vi "MCC 172 Noise.vi"() -> ()   [LabVIEW 2018]
uses:
  <vilib>/addons/_NISVFA/_Shared subVIs/Controls/svc_Window.ctl
  <vilib>/Analysis/5stat.llb/RMS (DBL).vi
  <vilib>/addons/Sound and Vibration/svt_Single Tone Measurements/SVT Idle Channel Noise (Time) (1 Ch).vi
  <vilib>/addons/_NISVFA/_Baseband FFT/SVFA Power Spectral Density (1 Ch).vi
  <vilib>/addons/_NISVFA/_Baseband FFT/SVFA Power Spectrum (1 Ch).vi
  <vilib>/addons/Sound and Vibration/svt_Single Tone Measurements/SoundVib_SingleTone.lvlib
  <vilib>/Analysis/NI_AALBase.lvlib
  <vilib>/Analysis/NI_AALPro.lvlib
  <vilib>/gmath/NI_Gmath.lvlib
panel:
  in  "?":bool
  in  "# of Averaging":u32=1
  in  "Tab Control":enum32{"Setup", "Plots"}(tab)
  in  "IEPE Power":bool
  out "Actual Sampling Rate":dbl
  in  "Desired Sampling Rate":dbl=51200.0
  in  "Server IP Address":string
  in  "Channel":u8
  out "averaging parameters":T1={"averaging mode"=enum."RMS averaging", "weighting mode"=enum."Linear", "number of averages"=1, "linear mode"=enum."Auto restart"} {"number of averages" min=1 step=1}
  out "Data":T2={"SVT"={"Noise (BW)"=6.638588448604977e-06, "SNR [dB]"=114.52750191336867, "Avg Noise Density"=8.304726164455459e-08, "Maximum Spur"={"Frequency"=10.6, "Spur Level"=3.655230318410738e-07}}, "Max Data"=-9.28286463022232e-05, "Data Range"=6.53464812785387e-05, "Mean(Offset)"=-0.00012652362230801374, "StdDev (Noise)"=7.540583269192075e-06, "RMS Value"=0.00012674812231162398, "Spread Value"=0.0}
  out "error out":errorcluster
  out "frequency range":T3={"start frequency"=10.0, "stop frequency"=6400.0} {"stop frequency" format="%.2f"; "start frequency" format="%.2f"}
  out "dt":dbl=7.8125e-05
  in  "Samples to read":u32=51200
  out "FFT Plot":cluster{"f0":dbl, "df":dbl, "magnitude":dbl[]}(graph)={"f0"=0.0, "df"=0.2, "magnitude"=[]}
  out "Histogram":dynamicdata(graph)
  out "Noise Density":cluster{"f0":dbl, "df":dbl, "magnitude":dbl[]}(graph)={"f0"=0.0, "df"=0.2, "magnitude"=[]}
  out "AI Data":waveform(dbl)(graph)
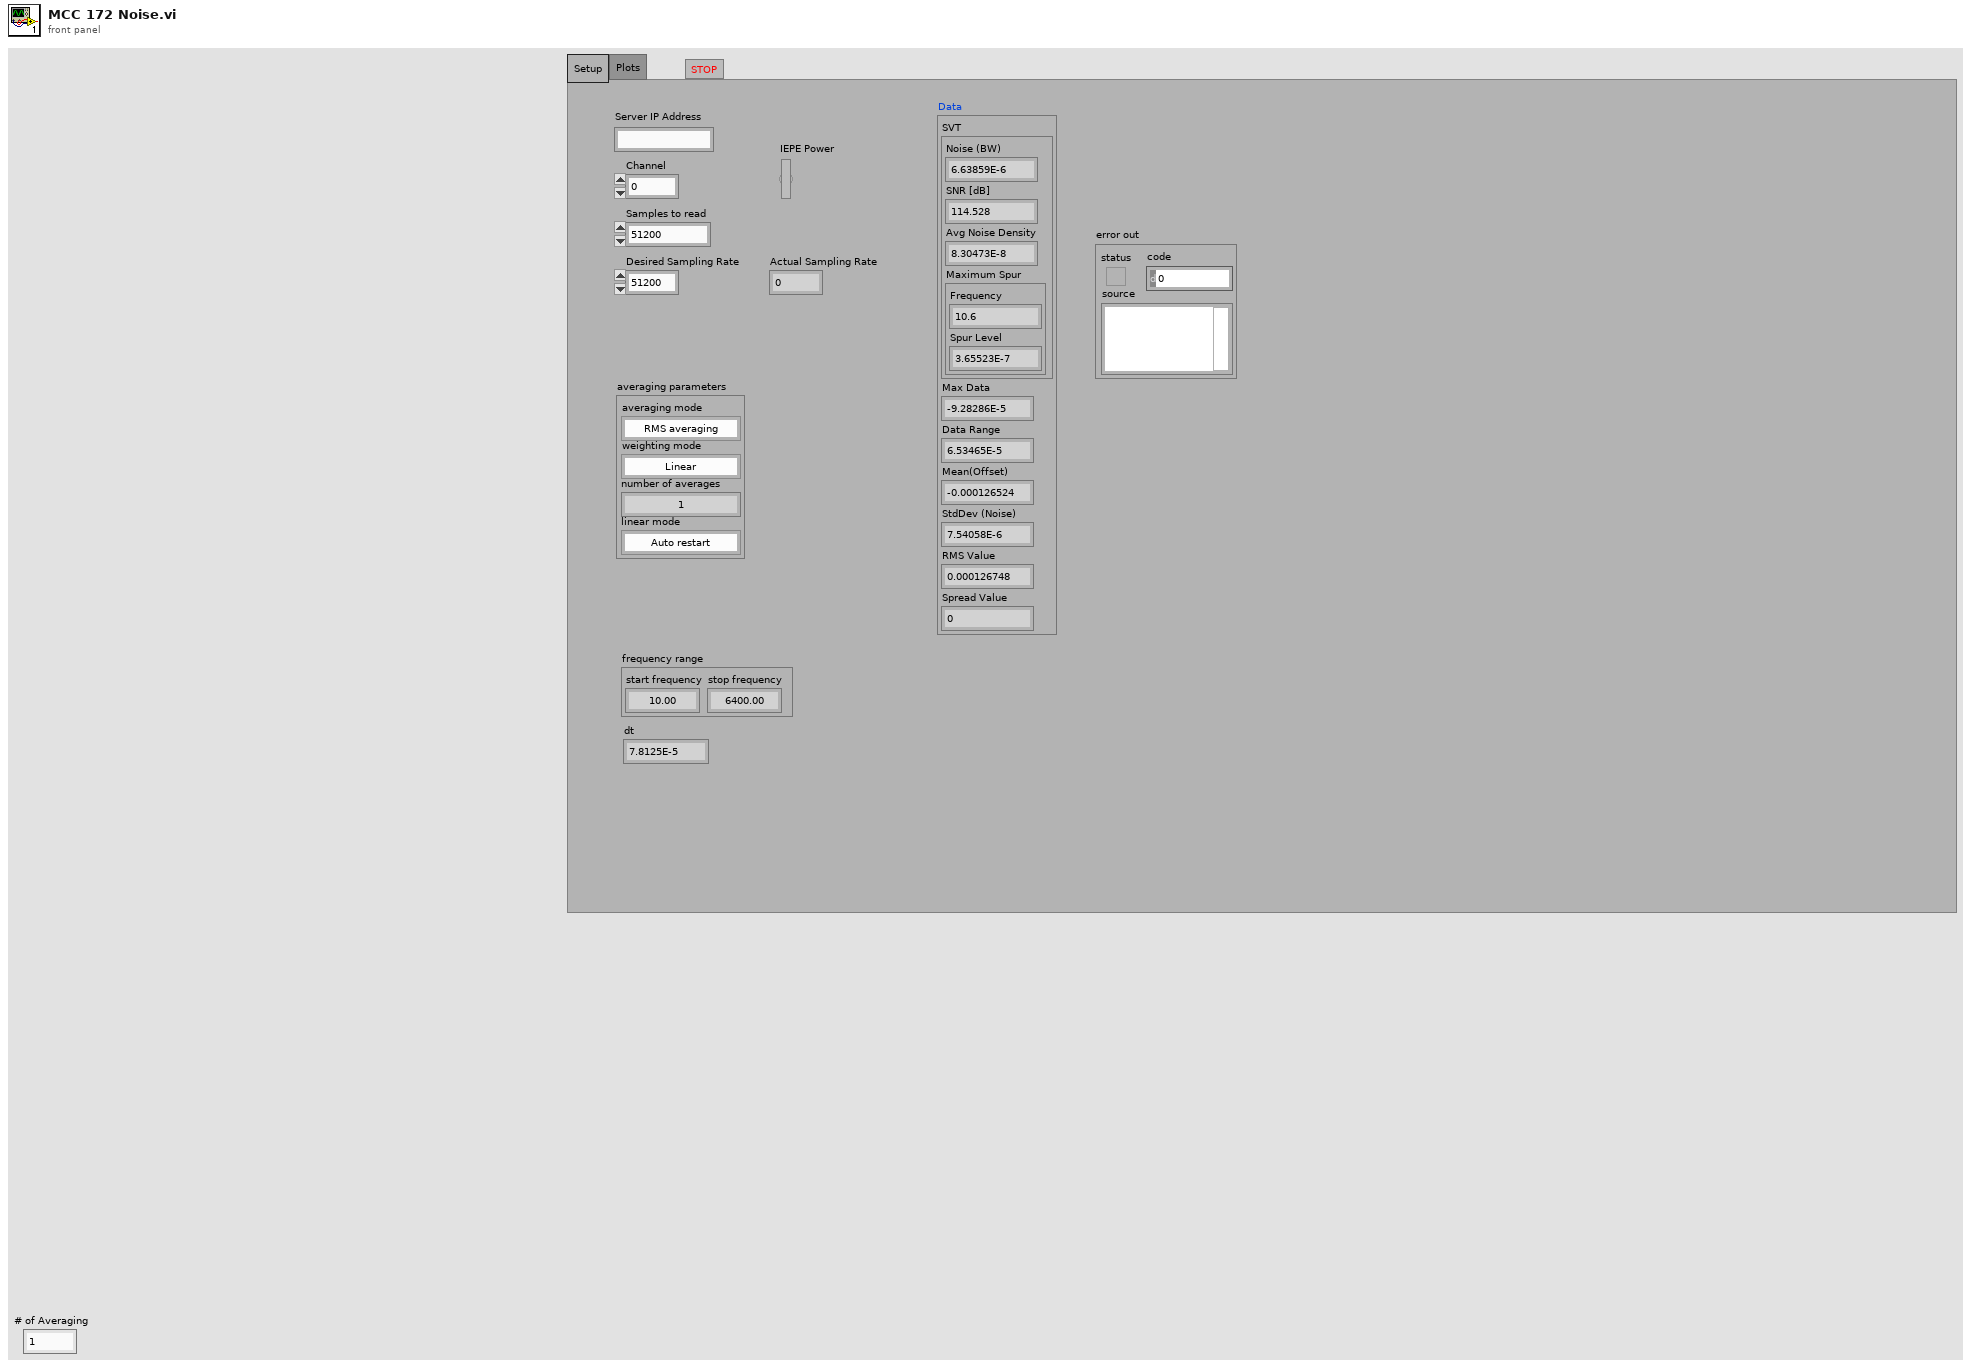
[diagram p1: front panel]
types:
  T1 = cluster{"averaging mode":enum16{"No averaging", "Vector averaging", "RMS averaging", "Peak hold"}, "weighting mode":enum16{"Linear", "Exponential"}, "number of averages":u32, "linear mode":enum16{"One shot", "Auto restart"}}
  T2 = cluster{"SVT":cluster{"Noise (BW)":dbl, "SNR [dB]":dbl, "Avg Noise Density":dbl, "Maximum Spur":cluster{"Frequency":dbl, "Spur Level":dbl}}, "Max Data":dbl, "Data Range":dbl, "Mean(Offset)":dbl, "StdDev (Noise)":dbl, "RMS Value":dbl, "Spread Value":dbl}
  T3 = cluster{"start frequency":dbl, "stop frequency":dbl}
  T4 = enum16{"No averaging", "Vector averaging", "RMS averaging", "Peak hold"}
  T5 = cluster{"idle channel noise units":enum16{"dB", "EU^2 rms"}}
  T6 = typedef "svc_Window.ctl" = u32
  T7 = cluster{dbl, "SNR [dB]":dbl, "average noise level [EU / sqrt(Hz)]":dbl, "maximum spur [EU rms]":cluster{"frequency":dbl, "value":dbl}}
  T8 = cluster{cluster{dbl, "SNR [dB]":dbl, "average noise level [EU / sqrt(Hz)]":dbl, "maximum spur [EU rms]":cluster{"frequency":dbl, "value":dbl}}, dbl, dbl, "mean":dbl, "standard deviation":dbl, "rms value":dbl, "spread value":dbl}
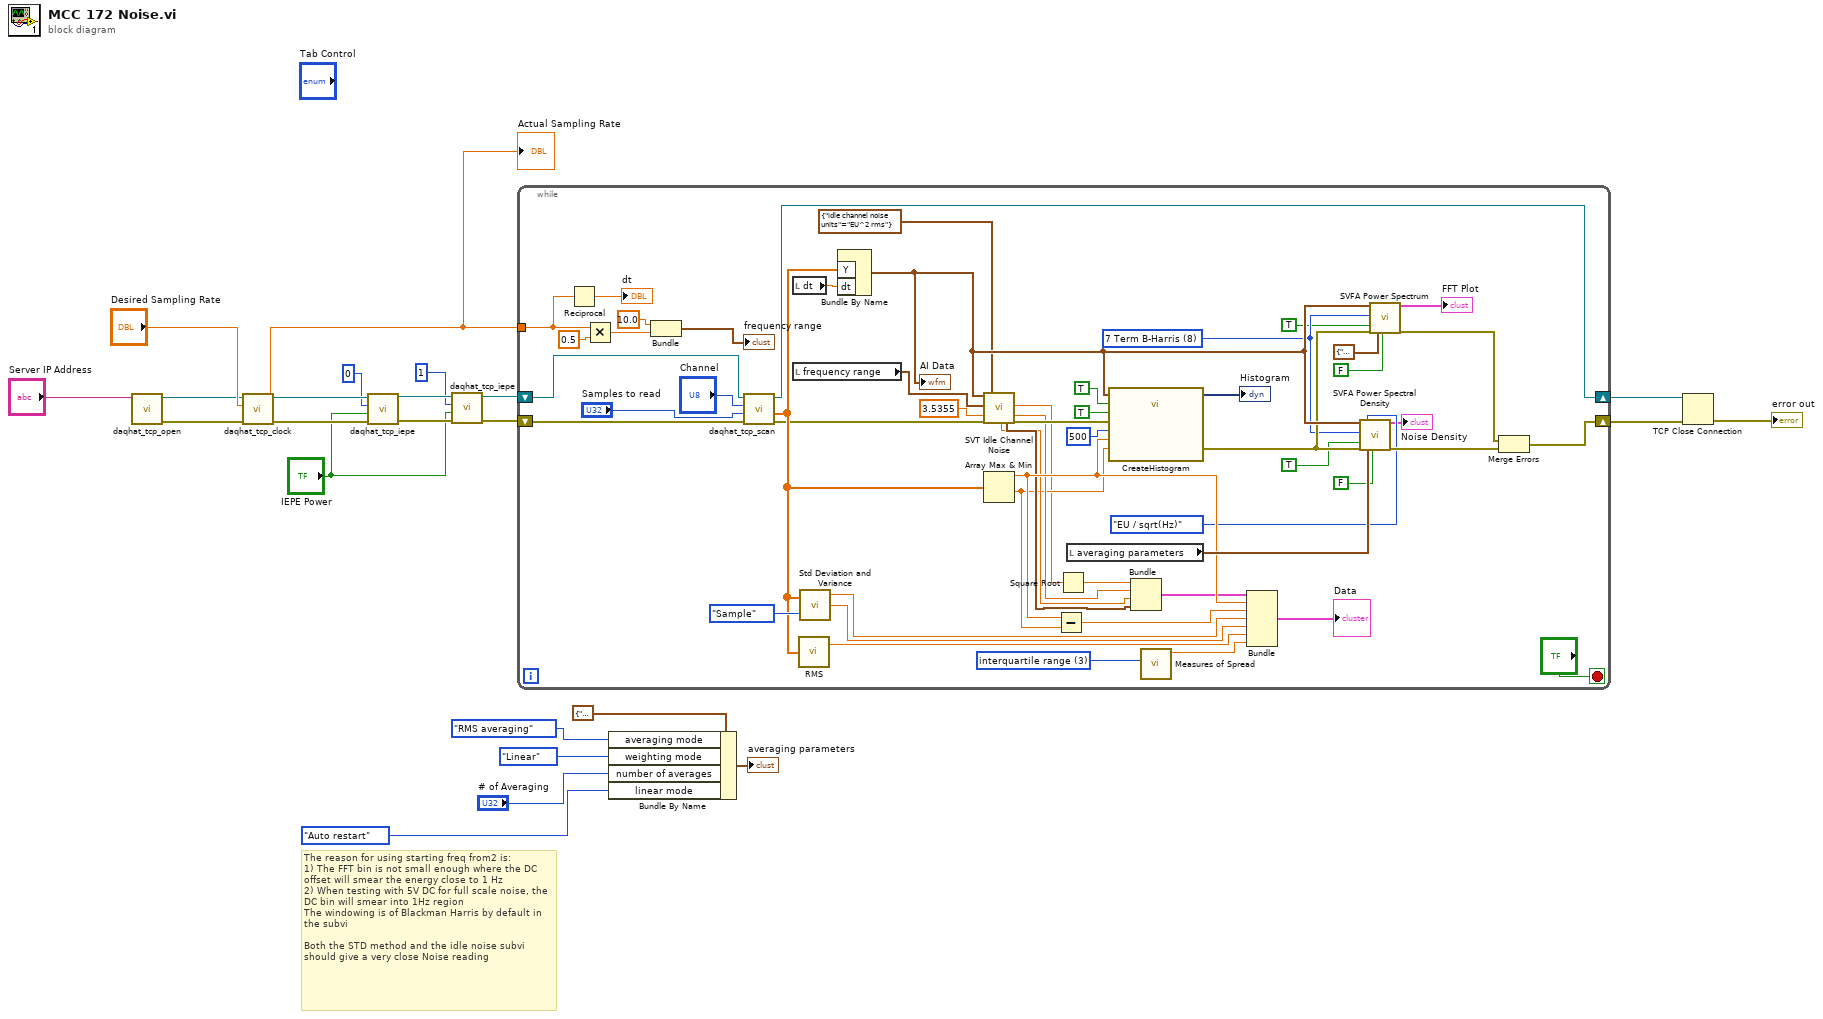
[diagram p0: block diagram]
diagram:
  # "The reason for using starting freq from2 is:\n1) The FFT bin is not small enough where the DC offset will smear the energy close to 1 Hz\n2) When testing with 5V DC for full scale noise, the DC bin will smear into 1Hz region\nThe windowing is of Blackman Harris by default in the subvi\n\nBoth the STD method and the idle noise subvi should give a very close Noise reading"
  n1 = call "daqhat_tcp_open.vi"("Server IP Address"="Server IP Address") -> ("error out"=w11:errorcluster, "TCP Network Connection out"=w10:refnum<k5>)  [unwired: 9 in]
  n2 = call "daqhat_tcp_clock.vi"("error in (no error)"=w11, "Desired frequency"="Desired Sampling Rate", "TCP network connection in"=w10) -> ("error out"=w8:errorcluster, "Set frequency"=w20:dbl, "TCP Network Connection out"=w9:refnum<k5>)  [unwired: 6 in]
  "Actual Sampling Rate" <- w20
  n3 = call "daqhat_tcp_iepe.vi"("error in (no error)"=w8, "IEPE Power"="IEPE Power", "Channel"=0, "TCP network connection in"=w9) -> ("error out"=w4:errorcluster, "TCP Network Connection out"=w3:refnum<k5>)  [unwired: 6 in]
  n4 = call "daqhat_tcp_iepe.vi"("error in (no error)"=w4, "IEPE Power"="IEPE Power", "Channel"=1, "TCP network connection in"=w3) -> ("error out"=w5:errorcluster, "TCP Network Connection out"=w6:refnum<k5>)  [unwired: 6 in]
  n5 = while {
    shift-right: [w37] -> w21
    shift-left: w5 -> [w42]
    shift-right: [w38] -> w23
    shift-left: w6 -> [w41]
    tunnel: w20 -> [w24]
    stop <- "?" stop-if-true
    w53 = T6 8 items=["None"=0, "Hanning"=1, "Hamming"=2, "Blackman-Harris"=3, "Exact Blackman"=4, "Blackman"=5, "Flat Top"=6, "4 Term B-Harris "=7, "7 Term B-Harris"=8, "Low Sidelobe"=9, "Force"=64, "Exponential"=65, "Blackman Nuttall"=11, "Triangle"=30, "Bartlett-Hanning"=31, "Bohman"=32, "Parzen"=33, "Welch"=34, "Kaiser"=60, "Dolph-Chebyshev"=61, "Gaussian"=62] ("window")
    w46 = 3 items=["standard deviation", "range", "mean absolute deviation", "interquartile range"] ("type")
    n6 = Reciprocal(x=w24) -> (1/x=→"dt":dbl)
    n7 = Multiply(x=w24, y=0.5) -> (x*y=w28:dbl)
    n8 = Bundle(10.0, w28) -> (→"frequency range":cluster{dbl, dbl})  [unwired: 1 in]
    n9 = call "daqhat_tcp_scan.vi"("error in (no error)"=w42, "Sample count"="Samples to read", "Analog channel"="Channel", "TCP network connection in"=w41) -> ("error out"=w39:errorcluster, "Sample data"=w40:dbl[], "TCP Network Connection out"=w38:refnum<k5>)  [unwired: 4 in, 1 out]
    n10 = local read "dt"() -> (w72:dbl)
    n11 = local read "frequency range"() -> (w73:T3)
    n12 = call-poly <vilib>:"RMS.vi"("X"=w40) -> ("rms value"=w68:dbl)  [unwired: 1 out]
    n13 = call <vilib>:"Std Deviation and Variance.vi"("X"=w40, "Weighting (Sample)"=enum16{"Sample", "Population"}."Sample") -> ("mean"=w66:dbl, "standard deviation"=w67:dbl)  [unwired: 1 out]
    n14 = Bundle By Name("Y"=w40, "dt"=w72) -> (w77:waveform(dbl))  [unwired: 1 in]
    "AI Data" <- w77
    n15 = call-poly <vilib>:"SVT Idle Channel Noise.vi"("scaled signal [EU]"=w77, "frequency range"=w73, "full-scale level [EU rms]"=3.5355, "error in (no error)"=w39, "desired units"=T5 {"idle channel noise units"=enum."EU^2 rms"}) -> ("average noise level [EU / sqrt(Hz)]"=w61:dbl, "maximum spur [EU rms]"=w62:cluster{"frequency":dbl, "value":dbl}, "idle channel noise"=w57:dbl, "SNR [dB]"=w60:dbl, "error out"=w70:errorcluster)  [unwired: 7 in, 3 out]
    n16 = Array Max & Min(array=w40) -> (max value=w64:dbl, min value=w58:dbl)  [unwired: 2 out]
    n17 = Subtract(x=w64, y=w58) -> (x-y=w65:dbl)
    n18 = Square Root(x=w57) -> (sqrt(x)=w59:dbl)
    n19 = local read "averaging parameters"() -> (w74:T1)
    n20 = call "CreateHistogram.vi"("Maximum Value"=w64, "Number of Bins"=500, "Minimum Value"=w58, "error in (no error)"=w70, "Reset"=TRUE, "Enable"=TRUE, "Signal"=w77) -> ("error out"=w71:errorcluster, "Histogram"=→"Histogram":dynamicdata)  [unwired: 3 in]
    n21 = Bundle(w59, "SNR [dB]"=w60, "average noise level [EU / sqrt(Hz)]"=w61, "maximum spur [EU rms]"=w62) -> (w63:T7)  [unwired: 1 in]
    n22 = call <vilib>:"Measures of Spread.vi"("type"=w46) -> ("spread value"=w69:dbl)  [unwired: 9 in, 1 out]
    n23 = Bundle(w63, w64, w65, "mean"=w66, "standard deviation"=w67, "rms value"=w68, "spread value"=w69) -> (→"Data":T8)  [unwired: 1 in]
    n24 = call-poly <vilib>:"SVFA Power Spectral Density.vi"("scaled signal [EU]"=w77, "window"=w53, "dB On (F)"=TRUE, "error in (no error)"=w71, "desired units"=enum16{"EU^2 / Hz", "EU / sqrt(Hz)"}."EU / sqrt(Hz)", "averaging parameters"=w74, "restart averaging (F)"=FALSE) -> ("power spectral density [EU^2 rms / Hz]"=→"Noise Density":cluster{"f0":dbl, "df":dbl, "magnitude":dbl[]}, "error out"=w76:errorcluster)  [unwired: 7 in, 4 out]
    n25 = call-poly <vilib>:"SVFA Power Spectrum.vi"("scaled signal [EU]"=w77, "window"=w53, "dB On (T)"=TRUE, "error in (no error)"=w71, "averaging parameters"=T1 {"averaging mode"=enum."No averaging", "weighting mode"=enum."Exponential", "number of averages"=10, "linear mode"=enum."One shot"}, "restart averaging (F)"=FALSE) -> ("power spectrum [dB EU]"=→"FFT Plot":cluster{"f0":dbl, "df":dbl, "magnitude":dbl[]}, "error out"=w75:errorcluster)  [unwired: 8 in, 4 out]
    n26 = Merge Errors(w75, w76) -> (w37:errorcluster)
  }
  n27 = Bundle By Name(cluster=T1 {"averaging mode"=enum."No averaging", "weighting mode"=enum."Exponential", "number of averages"=10, "linear mode"=enum."One shot"} ("averaging parameters"), "averaging mode"=T4."RMS averaging", "weighting mode"=enum16{"Linear", "Exponential"}."Linear", "number of averages"="# of Averaging", "linear mode"=enum16{"One shot", "Auto restart"}."Auto restart") -> (→"averaging parameters":T1)
  n28 = TCP Close Connection(connection ID=w23, error in (no error)=w21) -> (error out=→"error out":errorcluster)  [unwired: 1 in, 1 out]
